vi "Read Aerotech Controller.vi"(8 "error in (no error)":errorcluster, 11 "Gantry Class in":refnum<class "Gantry Class.lvclass">) -> (0 "error out":errorcluster, 2 "Aerotech Controller":refnum<k24>, 3 "Gantry Class out":refnum<class "Gantry Class.lvclass">)   [LabVIEW 2011, in "Gantry Class.lvclass"]
uses:
  Gantry Class.lvclass
  C:/Program Files/National Instruments/LabVIEW 2011/user.lib/aerotech/8.2/Bin/Aerotech.A3200.dll
  Program Files/National Instruments/LabVIEW 2011/user.lib/aerotech/8.2/Bin/Aerotech.A3200.dll
  Gantry Class.lvclass/Gantry Class.ctl
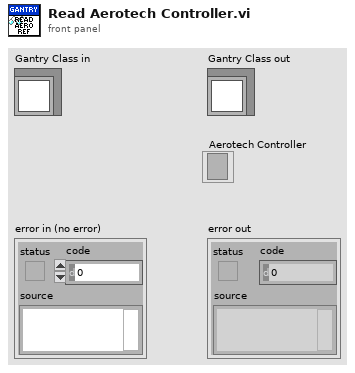
[diagram p1: front panel]
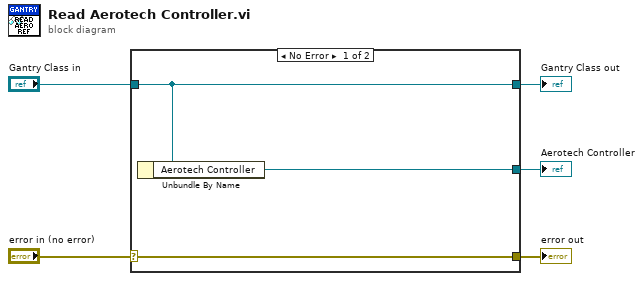
[diagram p0: block diagram]
diagram:
  n1 = case shown="No Error" "error in (no error)" {
    selector: "error in (no error)" -> [w8 w9]
    tunnel: [w8 w9] -> w4
    tunnel: [w7 w10] -> w2
    tunnel: "Gantry Class in" -> [w7 w10]
    tunnel: [w6 _] -> w1
    frame No Error {
      n2 = Unbundle By Name(w7) -> ("Aerotech Controller"=w6:refnum<k24>)
    }
    frame Error {
    }
  }
  "error out" <- w4
  "Gantry Class out" <- w2
  "Aerotech Controller" <- w1
